vi "GDC Befehl und Antwort.vi"(8 "error in (no error)":errorcluster caption="Fehler (Eingang, kein Fehler)", 9 "Daten":string[](array[string]), 10 "Befehl":string, 11 "VISA-Ressourcenname":refnum<visa-resource-name>) -> (0 "error out":errorcluster caption="Fehler (Ausgang)", 1 "Daten":string, 2 "Befehl":string, 3 "VISA-Ressourcenname (Ausgang)":refnum<visa-resource-name>)   [LabVIEW 2020, in "Linearisierung v2.lvlib" / "Gasteiler.lvlib" / "Horiba GDC.lvlib"]
uses:
  Horiba GDC.lvlib
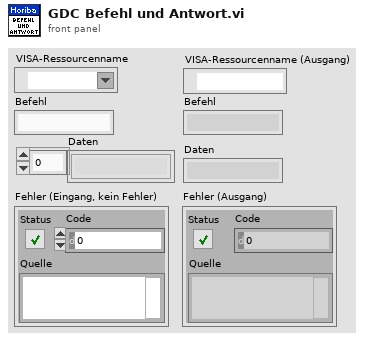
[diagram p1: front panel]
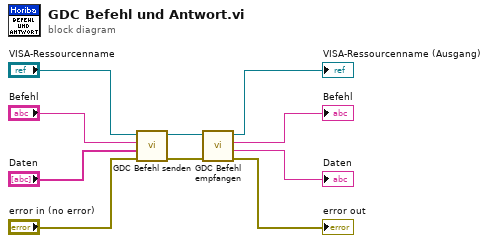
[diagram p0: block diagram]
diagram:
  n1 = call "GDC Befehl senden.vi"("error in (no error)"="error in (no error)", "Daten"="Daten", "Befehl"="Befehl", "VISA-Ressourcenname"="VISA-Ressourcenname") -> ("error out"=w8:errorcluster, "VISA-Ressourcenname (Ausgang)"=w9:refnum<visa-resource-name>)  [unwired: 6 in]
  n2 = call "GDC Befehl empfangen.vi"("error in (no error)"=w8, "VISA-Ressourcenname"=w9) -> ("error out"=→"error out":errorcluster, "Daten"=→"Daten":string, "Befehl"=→"Befehl":string, "VISA-Ressourcenname (Ausgang)"=→"VISA-Ressourcenname (Ausgang)":refnum<visa-resource-name>)  [unwired: 6 in]
